vi "Test Assert Equal Value and Type.vi"(8 "error in (no error)":errorcluster) -> (0 "error out":errorcluster)   [LabVIEW 2009]
uses:
  classes/Assert/Assert.lvclass
  classes/Test/Test.lvclass
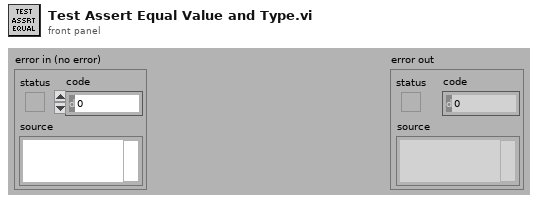
[diagram p1: front panel]
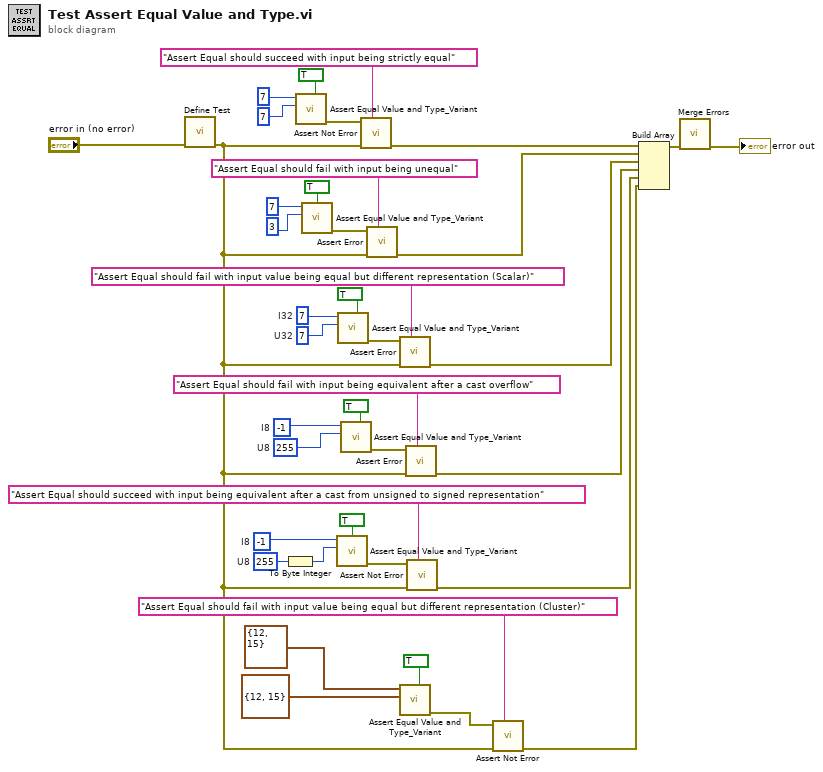
[diagram p0: block diagram]
diagram:
  w32 = u8 255  # U8
  w9 = i8 -1  # I8
  w13 = u8 255  # U8
  w14 = i8 -1  # I8
  w18 = u32 7  # U32
  w17 = 7  # I32
  n1 = call "Define Test.vi"("error in (no error)"="error in (no error)") -> ("error out"=w7:errorcluster)  [unwired: 10 in]
  n2 = To Byte Integer(number=w32) -> (8bit integer=w8:i8)
  n3 = call "Assert Equal Value and Type_Variant.vi"("Assert Only? (F)"=TRUE, "Y"=7, "X"=7) -> ("error out"=w30:errorcluster)  [unwired: 8 in]
  n4 = call "Assert Equal Value and Type_Variant.vi"("Assert Only? (F)"=TRUE, "Y"=3, "X"=7) -> ("error out"=w25:errorcluster)  [unwired: 8 in]
  n5 = call "Assert Equal Value and Type_Variant.vi"("Assert Only? (F)"=TRUE, "Y"=w8, "X"=w9) -> ("error out"=w10:errorcluster)  [unwired: 8 in]
  n6 = call "Assert Equal Value and Type_Variant.vi"("Assert Only? (F)"=TRUE, "Y"=w18, "X"=w17) -> ("error out"=w19:errorcluster)  [unwired: 8 in]
  n7 = call "Assert Equal Value and Type_Variant.vi"("Assert Only? (F)"=TRUE, "Y"=w13, "X"=w14) -> ("error out"=w15:errorcluster)  [unwired: 8 in]
  n8 = call "Assert Not Error.vi"("Label"="Assert Equal should succeed with input being strictly equal", "error in (no error)"=w7, "Not Error?"=w30) -> ("error out"=w37:errorcluster)  [unwired: 8 in]
  n9 = call "Assert Error.vi"("Label"="Assert Equal should fail with input being unequal", "error in (no error)"=w7, "Error?"=w25) -> ("error out"=w36:errorcluster)  [unwired: 8 in]
  n10 = call "Assert Error.vi"("Label"="Assert Equal should fail with input value being equal but different representation (Scalar)", "error in (no error)"=w7, "Error?"=w19) -> ("error out"=w22:errorcluster)  [unwired: 8 in]
  n11 = call "Assert Equal Value and Type_Variant.vi"("Assert Only? (F)"=TRUE, "Y"=cluster{"Width":u32, "U32":u32} {"Width"=12, "U32"=15} ("Bounds"), "X"=cluster{"Width":u32, "I32":i32} {"Width"=12, "I32"=15} ("Bounds")) -> ("error out"=w1:errorcluster)  [unwired: 8 in]
  n12 = call "Assert Error.vi"("Label"="Assert Equal should fail with input being equivalent after a cast overflow", "error in (no error)"=w7, "Error?"=w15) -> ("error out"=w21:errorcluster)  [unwired: 8 in]
  n13 = call "Assert Not Error.vi"("Label"="Assert Equal should succeed with input being equivalent after a cast from unsigned to signed representation", "error in (no error)"=w7, "Not Error?"=w10) -> ("error out"=w20:errorcluster)  [unwired: 8 in]
  n14 = call "Assert Not Error.vi"("Label"="Assert Equal should fail with input value being equal but different representation (Cluster)", "error in (no error)"=w7, "Not Error?"=w1) -> ("error out"=w6:errorcluster)  [unwired: 8 in]
  n15 = Build Array(w37, w36, w22, w21, w20, w6) -> (w35:errorcluster[])
  n16 = call <vilib>:"Merge Errors.vi"("error array in"=w35) -> ("error out"=→"error out":errorcluster)  [unwired: 6 in]
